vi "serialization test.vi"() -> ()   [LabVIEW 2013, in "std eng tests.lvlib"]
uses:
  std eng tests.lvlib
  Runtime/Standard Engine Runtime.lvclass
  <vilib>/NI/Tag Bus Module Framework/channel/channel classification.ctl
  Configuration/Module Decimation.ctl
  Configuration/Supported Timing Sources.ctl
  testmodule/execution/testmod runtime.lvclass
  testmodule/configuration/testmod configuration.lvclass
  <vilib>/NI/Tag Bus/tag/Data Type.ctl
  Configuration/Module Error Configuration.ctl
  Configuration/Error Actions By Category.ctl
  <vilib>/NI/Tag Bus Module Framework/runtime/error classification.ctl
  Configuration/Error Actions.ctl
  Configuration/timing reporting tags.ctl
  Configuration/Standard Engine Configuration.lvclass
  Configuration/Standard Engine Configuration.lvclass/Standard Engine Configuration.ctl
  <vilib>/NI/Tag Bus/tag/tag descriptor.lvclass/tag descriptor.ctl
  Configuration/Write Timing Source Type.vi
  Configuration/Read Master Timing Module.vi
  Configuration/Read Module Specific Configuration.vi
  Configuration/Read Processor.vi
  Configuration/Read timing policy.vi
  Configuration/Read Timing Source Type.vi
  Configuration/Write Timing Source dt.vi
  <vilib>/NI/Tag Bus/tag/validate default value.vi
  Configuration/Find Module Specific Config.vi
  <vilib>/Utility/error.llb/Error Cluster From Error Code.vi
  Configuration/Read Timing Source dt.vi
  <vilib>/NI/Tag Bus/tag/tag descriptor.lvclass
  <vilib>/NI/Tag Bus Module Framework/channel/TBM channel.lvclass
  <vilib>/NI/Module Execution Interface/Engine Configuration/engine configuration.lvclass
  <vilib>/NI/Tag Bus Module Framework/runtime/TBM module execution interface.lvclass
panel:
  out "serialization ok 7":bool
  out "serialization ok 6":bool
  out "serialization ok 5":bool
  out "serialization ok 4":bool
  out "serialization ok 3":bool
  out "serialization ok 2":bool
  out "serialization ok":bool
  out "errrrr":errorcluster
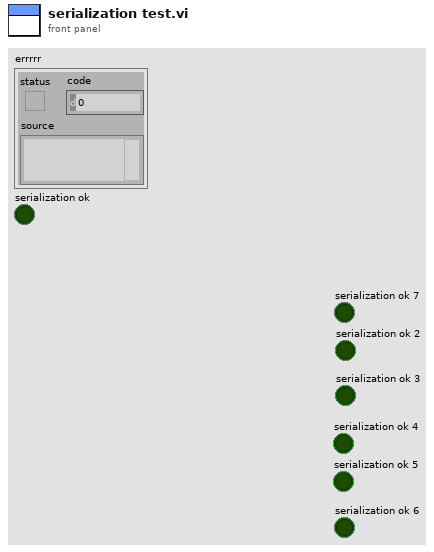
[diagram p1: front panel]
types:
  T1 = typedef "Standard Engine Configuration.lvclass/timing reporting tags.ctl" = cluster{"late index (bool)":string, "late count index (U32)":string, "current dt (U32)":string}
  T2 = typedef "tag bus.lvlib/tag descriptor.lvclass/Data Type.ctl" = enum16{"Double", "Single", "I64", "I32", "I16", "I8", "U64", "U32", "U16", "U8", "Boolean", "String", "Array of Double", "Array of Single", "Array of I64", "Array of I32", "Array of I16", "Array of I8", "Array of U64", "Array of U32", "Array of U16", "Array of U8", "Array of Boolean", "Array of String"}
  T3 = typedef "TBM channel.lvclass/channel classification.ctl" = enum16{"input data", "output data", "processing parameter", "processing result"}
  T4 = typedef "Standard Engine Configuration.lvclass/Error Actions By Category.ctl" = cluster{"error classification":T5, "Error Actions":T6[]}
  T5 = typedef "TBM module execution interface.lvclass/error classification.ctl" = enum16{"unknown", "none", "trivial", "recoverable", "critical"}
  T6 = typedef "Standard Engine Configuration.lvclass/Error Actions.ctl" = enum16{"Clear", "Notify", "Stop Component", "Stop Engine", "Safe State", "Attempt Recovery"}
  T7 = typedef "Standard Engine Configuration.lvclass/Module Error Configuration.ctl" = cluster{"Module Error Configuration":T4[]}
  T8 = typedef "Standard Engine Configuration.lvclass/Supported Timing Sources.ctl" = enum16{"Use Module Timing Source", "1 kHz Clock", "1 MHz Clock", "Synchronize to Scan Engine"}
  T9 = typedef "Standard Engine Configuration.lvclass/Module Decimation.ctl" = cluster{"Decimation":u16, "Offset":u16}
  T10 = typedef "Standard Engine Configuration.lvclass/Module Specific Configuration.ctl" = cluster{"Module ID":string, "Module Decimation":T9, "Module Error Configuration":T7, "execution order priority":i32, "async?":bool, "error tag":string}
  T11 = typedef "Standard Engine Configuration.lvclass/timing policy.ctl" = enum16{"strict determinism", "nonblocking", "nondeterministic inline"}
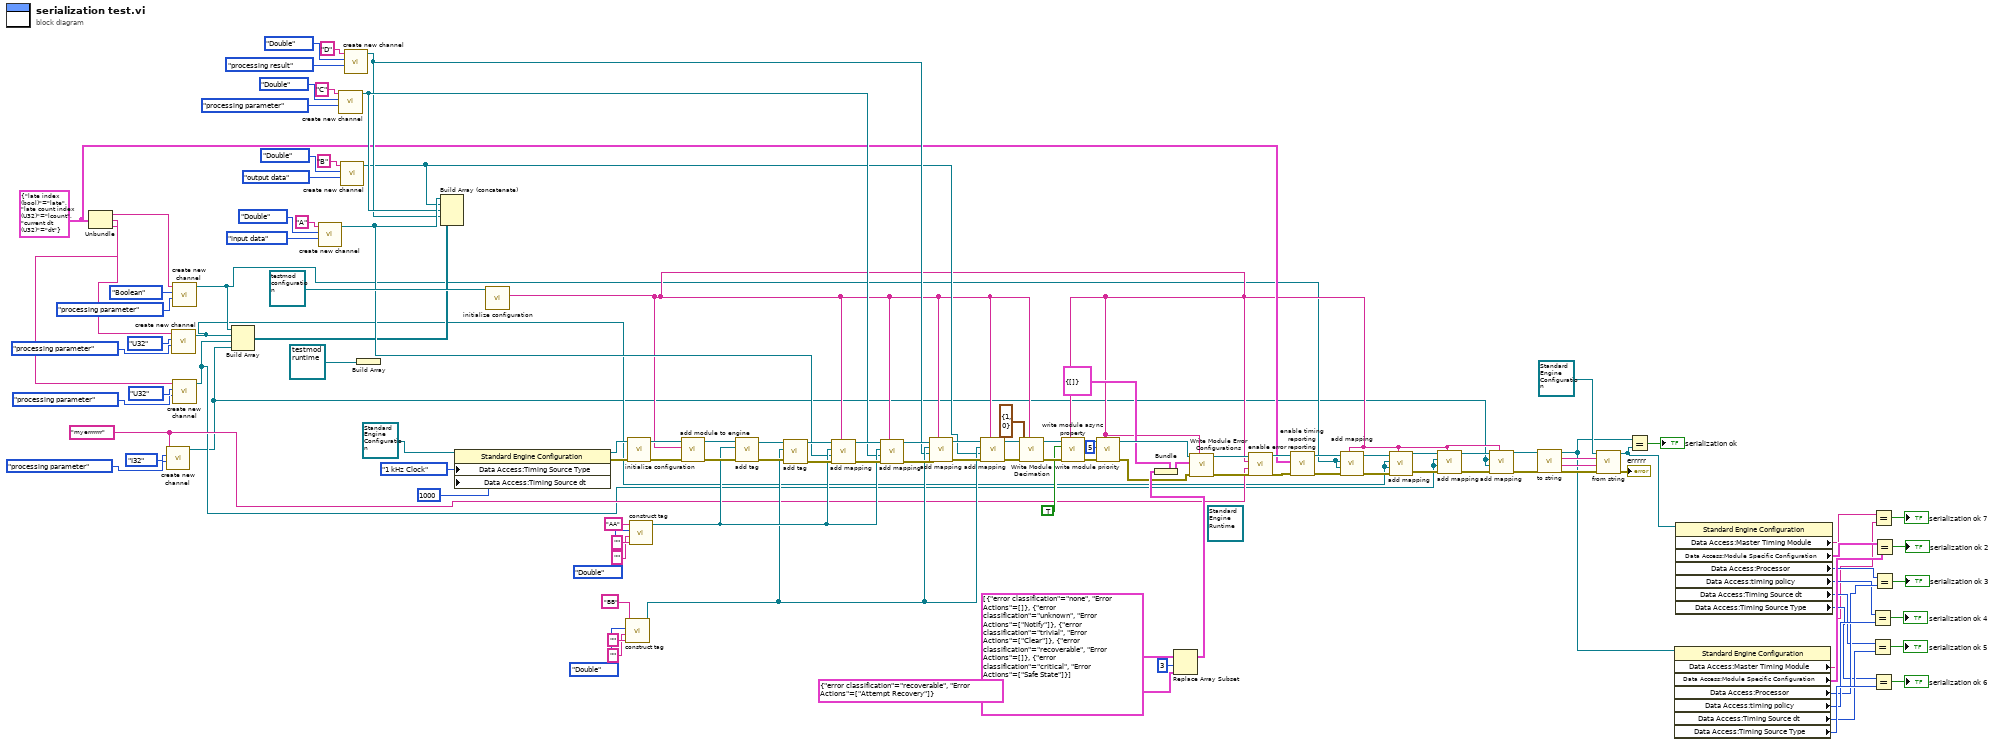
[diagram p0: block diagram]
diagram:
  w42 = T1 {"late index (bool)"="late", "late count index (U32)"="lcount", "current dt (U32)"="dt"} ("timing reporting")
  w43 = "myerrrrrrr" ("channel name")
  (unwired) refnum<class "Standard Engine Runtime.lvclass"> refnum ("Standard Engine Runtime")
  n1 = Unbundle(w42) -> ("late index (bool)"=w49:string, "late count index (U32)"=w48:string, "current dt (U32)"=w47:string)
  n2 = call <vilib>:"create new channel.vi"("channel classification"=channel_classification."processing parameter", "data type"=Data_Type."I32", "channel name"=w43) -> ("channel"=w29:refnum<class "TBM channel.lvclass">)  [unwired: 8 in]
  n3 = call <vilib>:"create new channel.vi"("channel classification"=channel_classification."processing parameter", "data type"=Data_Type."U32", "channel name"=w48) -> ("channel"=w31:refnum<class "TBM channel.lvclass">)  [unwired: 8 in]
  n4 = call <vilib>:"create new channel.vi"("channel classification"=channel_classification."processing parameter", "data type"=Data_Type."Boolean", "channel name"=w49) -> ("channel"=w32:refnum<class "TBM channel.lvclass">)  [unwired: 8 in]
  n5 = call <vilib>:"create new channel.vi"("channel classification"=channel_classification."processing parameter", "data type"=Data_Type."U32", "channel name"=w47) -> ("channel"=w30:refnum<class "TBM channel.lvclass">)  [unwired: 8 in]
  n6 = Build Array(w32, w31, w30, w29) -> (w44:refnum<class "TBM channel.lvclass">[])
  n7 = call <vilib>:"create new channel.vi"("channel classification"=channel_classification."input data", "data type"=Data_Type."Double", "channel name"="A") -> ("channel"=w71:refnum<class "TBM channel.lvclass">)  [unwired: 8 in]
  n8 = call <vilib>:"create new channel.vi"("channel classification"=channel_classification."processing parameter", "data type"=Data_Type."Double", "channel name"="C") -> ("channel"=w70:refnum<class "TBM channel.lvclass">)  [unwired: 8 in]
  n9 = call <vilib>:"create new channel.vi"("channel classification"=channel_classification."output data", "data type"=Data_Type."Double", "channel name"="B") -> ("channel"=w68:refnum<class "TBM channel.lvclass">)  [unwired: 8 in]
  n10 = call <vilib>:"create new channel.vi"("channel classification"=channel_classification."processing result", "data type"=Data_Type."Double", "channel name"="D") -> ("channel"=w69:refnum<class "TBM channel.lvclass">)  [unwired: 8 in]
  n11 = Build Array(refnum<class "testmod runtime.lvclass"> refnum ("CVT runtime")) -> ()  [unwired: 1 out]
  n12 = Build Array (concatenate)(w71, w68, w70, w69, w44) -> ()  [unwired: 1 out]
  n13 = property class="Standard Engine Configuration"(reference=refnum<class "Standard Engine Configuration.lvclass"> refnum ("Standard Engine Configuration"), "Data Access:Timing Source Type"=Supported_Timing_Sources."1 kHz Clock" ("Timing Source Type"), "Data Access:Timing Source dt"=u32 1000 ("Timing Source dt")) -> (reference out=w100:refnum<class "Standard Engine Configuration.lvclass">, error out=w102:errorcluster)  [unwired: 1 in]
  n14 = call-dynamic "initialize configuration.vi"("configuration in"=refnum<class "testmod configuration.lvclass"> refnum ("CVT configuration")) -> ("instance identifier"=w33:string)  [unwired: 8 in, 2 out]
  n15 = call <vilib>:"construct tag.vi"("raw default"="", "metadata"="", "data type"=Data_Type."Double", "name"="BB") -> ("system tag out"=w72:refnum<class "tag descriptor.lvclass">)  [unwired: 6 in, 1 out]
  n16 = call-dynamic "initialize configuration.vi"("error in"=w102, "configuration in"=w100) -> ("error out"=w113:errorcluster, "configuration out"=w112:refnum<class "Standard Engine Configuration.lvclass">)  [unwired: 7 in, 1 out]
  n17 = call <vilib>:"construct tag.vi"("raw default"="", "metadata"="", "data type"=Data_Type."Double", "name"="AA") -> ("system tag out"=w73:refnum<class "tag descriptor.lvclass">)  [unwired: 6 in, 1 out]
  n18 = call-dynamic "add module to engine.vi"("error in"=w113, "module ID"=w33, "Standard Engine Configuration in"=w112) -> ("error out"=w115:errorcluster, "Standard Engine Configuration out"=w114:refnum<class "Standard Engine Configuration.lvclass">)  [unwired: 7 in]
  n19 = call <vilib>:"add tag.vi"("error in"=w115, "tag descriptor"=w73, "engine configuration in"=w114) -> ("error out"=w88:errorcluster, "engine configuration out"=w89:refnum<class "Standard Engine Configuration.lvclass">)  [unwired: 7 in]
  n20 = call <vilib>:"add tag.vi"("error in"=w88, "tag descriptor"=w72, "engine configuration in"=w89) -> ("error out"=w87:errorcluster, "engine configuration out"=w75:refnum<class "Standard Engine Configuration.lvclass">)  [unwired: 7 in]
  n21 = call <vilib>:"add mapping.vi"("owner ID"=w33, "error in"=w87, "channel"=w71, "tag descriptor"=w73, "engine configuration"=w75) -> ("error out"=w76:errorcluster, "engine configuration out"=w74:refnum<class "Standard Engine Configuration.lvclass">)  [unwired: 5 in]
  n22 = call <vilib>:"add mapping.vi"("owner ID"=w33, "error in"=w76, "channel"=w70, "tag descriptor"=w73, "engine configuration"=w74) -> ("error out"=w78:errorcluster, "engine configuration out"=w77:refnum<class "Standard Engine Configuration.lvclass">)  [unwired: 5 in]
  n23 = call <vilib>:"add mapping.vi"("owner ID"=w33, "error in"=w78, "channel"=w69, "tag descriptor"=w72, "engine configuration"=w77) -> ("error out"=w117:errorcluster, "engine configuration out"=w116:refnum<class "Standard Engine Configuration.lvclass">)  [unwired: 5 in]
  n24 = call <vilib>:"add mapping.vi"("owner ID"=w33, "error in"=w117, "channel"=w68, "tag descriptor"=w72, "engine configuration"=w116) -> ("error out"=w108:errorcluster, "engine configuration out"=w109:refnum<class "Standard Engine Configuration.lvclass">)  [unwired: 5 in]
  n25 = call "Write Module Decimation.vi"("Module ID"=w33, "error in"=w108, "Module Decimation"=T9 {"Decimation"=1, "Offset"=0}, "Standard Engine Repo Data in"=w109) -> ("error out"=w110:errorcluster, "Standard Engine Repo Data out"=w111:refnum<class "Standard Engine Configuration.lvclass">)  [unwired: 6 in]
  n26 = call "write module async property.vi"("Module ID"=w33, "error in"=w110, "async?"=TRUE, "Standard Engine Repo Data in"=w111) -> ("error out"=w107:errorcluster, "Standard Engine Repo Data out"=w106:refnum<class "Standard Engine Configuration.lvclass">)  [unwired: 6 in]
  n27 = call "write module priority.vi"("Module ID"=w33, "error in"=w107, "execution order priority"=5, "Standard Engine Repo Data in"=w106) -> ("error out"=w56:errorcluster, "Standard Engine Repo Data out"=w67:refnum<class "Standard Engine Configuration.lvclass">)  [unwired: 6 in]
  n28 = Replace Array Subset(array=T4[] [{"error classification"=enum."none", "Error Actions"=[]}, {"error classification"=enum."unknown", "Error Actions"=[enum."Notify"]}, {"error classification"=enum."trivial", "Error Actions"=[enum."Clear"]}, {"error classification"=enum."recoverable", "Error Actions"=[]}, {"error classification"=enum."critical", "Error Actions"=[enum."Safe State"]}] ("Module Error Configuration"), new element=T4 {"error classification"=enum."recoverable", "Error Actions"=[enum."Attempt Recovery"]} ("Error Actions By Category"), index=3) -> (w63:T4[])
  n29 = Bundle(cluster=T7 {"Module Error Configuration"=[]} ("Module Error Configuration"), "Module Error Configuration"=w63) -> (w65:T7)
  n30 = call "Write Module Error Configurations.vi"("Module ID"=w33, "error in"=w56, "Module Error Configuration"=w65, "Standard Engine Repo Data in"=w67) -> ("error out"=w57:errorcluster, "Standard Engine Repo Data out"=w60:refnum<class "Standard Engine Configuration.lvclass">)  [unwired: 6 in]
  n31 = call "enable error reporting.vi"("error in"=w57, "tag"=w43, "module ID"=w33, "Standard Engine Configuration in"=w60) -> ("error out"=w58:errorcluster, "Standard Engine Configuration out"=w59:refnum<class "Standard Engine Configuration.lvclass">)  [unwired: 6 in]
  n32 = call "enable timing reporting.vi"("error in"=w58, "timing reporting"=w42, "Standard Engine Configuration in"=w59) -> ("error out"=w34:errorcluster, "Standard Engine Configuration out"=w35:refnum<class "Standard Engine Configuration.lvclass">)  [unwired: 7 in]
  n33 = call <vilib>:"add mapping.vi"("owner ID"=w33, "error in"=w34, "channel"=w32, "tag descriptor"=w32, "engine configuration"=w35) -> ("error out"=w40:errorcluster, "engine configuration out"=w41:refnum<class "Standard Engine Configuration.lvclass">)  [unwired: 5 in]
  n34 = call <vilib>:"add mapping.vi"("owner ID"=w33, "error in"=w40, "channel"=w31, "tag descriptor"=w31, "engine configuration"=w41) -> ("error out"=w38:errorcluster, "engine configuration out"=w39:refnum<class "Standard Engine Configuration.lvclass">)  [unwired: 5 in]
  n35 = call <vilib>:"add mapping.vi"("owner ID"=w33, "error in"=w38, "channel"=w30, "tag descriptor"=w30, "engine configuration"=w39) -> ("error out"=w36:errorcluster, "engine configuration out"=w37:refnum<class "Standard Engine Configuration.lvclass">)  [unwired: 5 in]
  n36 = call <vilib>:"add mapping.vi"("owner ID"=w33, "error in"=w36, "channel"=w29, "tag descriptor"=w29, "engine configuration"=w37) -> ("error out"=w27:errorcluster, "engine configuration out"=w26:refnum<class "Standard Engine Configuration.lvclass">)  [unwired: 5 in]
  n37 = call-dynamic "to string.vi"("error in"=w27, "Standard Engine Repo Data in"=w26) -> ("error out"=w28:errorcluster, "data"=w24:string, "version"=w25:string, "Standard Engine Repo Data out"=w19:refnum<class "Standard Engine Configuration.lvclass">)  [unwired: 6 in]
  n38 = call-dynamic "from string.vi"("error in"=w28, "data"=w24, "version"=w25, "Standard Engine Repo Data in"=refnum<class "Standard Engine Configuration.lvclass"> refnum ("Standard Engine Configuration")) -> ("error out"=→"errrrr":errorcluster, "Standard Engine Repo Data out"=w20:refnum<class "Standard Engine Configuration.lvclass">)  [unwired: 6 in]
  n39 = Equal?(x=w19, y=w20) -> (x = y?=→"serialization ok":bool)
  n40 = property class="Standard Engine Configuration"(reference=w19) -> ("Data Access:Master Timing Module"=w1:string, "Data Access:Module Specific Configuration"=w9:T10[], "Data Access:Processor"=w10:i32, "Data Access:timing policy"=w11:T11, "Data Access:Timing Source dt"=w12:u32, "Data Access:Timing Source Type"=w13:T8)  [unwired: 1 in, 2 out]
  n41 = property class="Standard Engine Configuration"(reference=w20) -> ("Data Access:Master Timing Module"=w2:string, "Data Access:Module Specific Configuration"=w8:T10[], "Data Access:Processor"=w7:i32, "Data Access:timing policy"=w6:T11, "Data Access:Timing Source dt"=w5:u32, "Data Access:Timing Source Type"=w4:T8)  [unwired: 1 in, 2 out]
  n42 = Equal?(x=w6, y=w11) -> (x = y?=→"serialization ok 4":bool)
  n43 = Equal?(x=w5, y=w12) -> (x = y?=→"serialization ok 5":bool)
  n44 = Equal?(x=w2, y=w1) -> (x = y?=→"serialization ok 7":bool)
  n45 = Equal?(x=w4, y=w13) -> (x = y?=→"serialization ok 6":bool)
  n46 = Equal?(x=w8, y=w9) -> (x = y?=→"serialization ok 2":bool)
  n47 = Equal?(x=w7, y=w10) -> (x = y?=→"serialization ok 3":bool)
